vi "Send Parent -  SEND - Triggered Event.vi"(7 "Message Priority (Normal)":T1=enum."Normal", 8 "error in (no error)":errorcluster, 10 "Actor_Interface.lvlib:Interface_Class.lvclass":refnum<class "Interface_Class.lvclass">=refnum, 11 "Message Enqueuer":refnum<class "Message Enqueuer.lvclass">) -> (0 "error out":errorcluster, 3 "Message Enqueuer out":refnum<class "Message Enqueuer.lvclass">)   [LabVIEW 2023, in "Actor_Parent.lvlib" / "Parent -  SEND - Triggered Event Msg.lvclass"]
doc: "This VI sends the message to an actor."
uses:
  Parent -  SEND - Triggered Event Msg.lvclass
  <vilib>/ActorFramework/Message Enqueuer/Message Enqueuer.lvclass
  C:/Program Files (x86)/National Instruments/LabVIEW 2023/vi.lib/ActorFramework/Message/Message.lvclass
  C:/Users/rodri/LabVIEW_Labs/LabVIEW_GitHub/LV-AF-Project/AF_Architecture/Message_Distributor/Parent_Class Messages/Parent -  SEND - Triggered Event Msg/Parent -  SEND - Triggered Event Msg.lvclass
  <vilib>/ActorFramework/Message Enqueuer/Message Priority.ctl
  Interface_Class/Interface_Class.lvclass
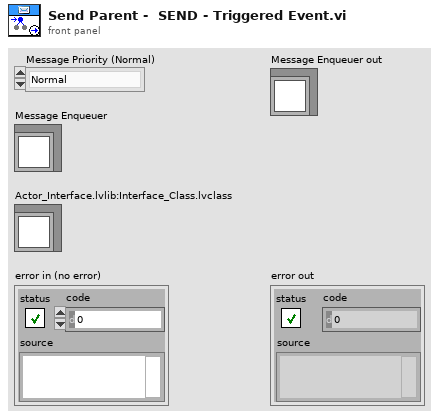
[diagram p1: front panel]
types:
  T1 = typedef "Actor Framework.lvlib/Message Enqueuer.lvclass/Message Priority.ctl" = enum16{"Low", "Normal", "High"}
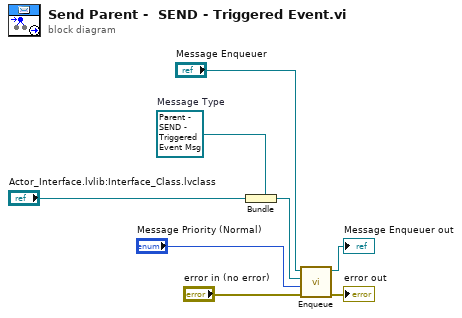
[diagram p0: block diagram]
diagram:
  w5 = refnum<class "Parent -  SEND - Triggered Event Msg.lvclass"> refnum  # Message Type
  n1 = Bundle(cluster=w5, "Actor_Interface.lvlib:Interface_Class.lvclass") -> (w4:refnum<class "Parent -  SEND - Triggered Event Msg.lvclass">)
  n2 = call <vilib>:"Enqueue.vi"("error in (no error)"="error in (no error)", "Message Priority (Normal)"="Message Priority (Normal)", "Message"=w4, "Message Enqueuer in"="Message Enqueuer") -> ("error out"=→"error out":errorcluster, "Message Enqueuer out"=→"Message Enqueuer out":refnum<class "Message Enqueuer.lvclass">)  [unwired: 6 in]
